vi "Check_Execution_Row.vi"(0 "Execution Row":T1 {"Carrier_2 Q (l/min)" format="%#.2f"; "Row Duration (mins)" format="%#.1f"; "Row No" min=0; "Trace Gas Concentration (%)" min=0.0 format="%#_4f"; "Carrier_1 Q (l/min)" format="%#.2f"; "Tunnel Speed" format="%#.2f"; "Start X" format="%#.2f"; "Start Y" format="%#.2f"; "Start Z" format="%#.2f"; "End X" format="%#.2f"; "End Y" format="%#.2f"; "End Z" format="%#.2f"; "Averaging time (min)" min=0.0 format="%#.2f"}, 1 "Earlier Filenames":path[](array[path]), 3 "Synchronization Start No":i32=1 min=1 max=100, 4 "Row Index":i32, 5 "Max Tunnel Speed":dbl format="%.2f") -> (6 "Edited Row":bool, 7 "Execution Row Out":T1 {"Carrier_2 Q (l/min)" format="%#.2f"; "Row Duration (mins)" format="%#.1f"; "Row No" min=0; "Trace Gas Concentration (%)" min=0.0 format="%#_4f"; "Carrier_1 Q (l/min)" format="%#.2f"; "Tunnel Speed" format="%#.2f"; "Start X" format="%#.2f"; "Start Y" format="%#.2f"; "Start Z" format="%#.2f"; "End X" format="%#.2f"; "End Y" format="%#.2f"; "End Z" format="%#.2f"; "Averaging time (min)" min=0.0 format="%#.2f"}, 9 "Continue?":bool, 10 "Error Comments":string)   [LabVIEW 2015]
uses:
  Traverse_cluster.ctl
  Spacing.ctl
  Controls/Multi_run_mode.ctl
  Controls/User_Specific_mode.ctl
  Controls/Home.ctl
  Controls/Tunnel_Coordinates.ctl
  ADAM Client/Sub VIs/ADAM Controls/Channel_names.ctl
  Globals/Extra_Commands_Global.vi
  Globals/Constants_global.vi
  Globals/Trav_pos_global.vi
panel:
  out "Traverse line Out":T1 {"Carrier_2 Q (l/min)" format="%#.2f"; "Row Duration (mins)" format="%#.1f"; "Row No" min=0; "Trace Gas Concentration (%)" min=0.0 format="%#_4f"; "Carrier_1 Q (l/min)" format="%#.2f"; "Tunnel Speed" format="%#.2f"; "Start X" format="%#.2f"; "Start Y" format="%#.2f"; "Start Z" format="%#.2f"; "End X" format="%#.2f"; "End Y" format="%#.2f"; "End Z" format="%#.2f"; "Averaging time (min)" min=0.0 format="%#.2f"}
  out "Fixed Axis":bool[](array[boolean])
  out "Filenames":string[](array[string])
  out "Current Sync Number":i32
  out "Checks":string[](array[string])
  in  "Edit in Excel":bool
  in  "OK":bool
  # "X           Y            Z"
  # "Start"
  # "End"
  # "X           Y            Z"
  # "Start"
  # "End"
  # "X           Y            Z"
  # "Start"
  # "End"
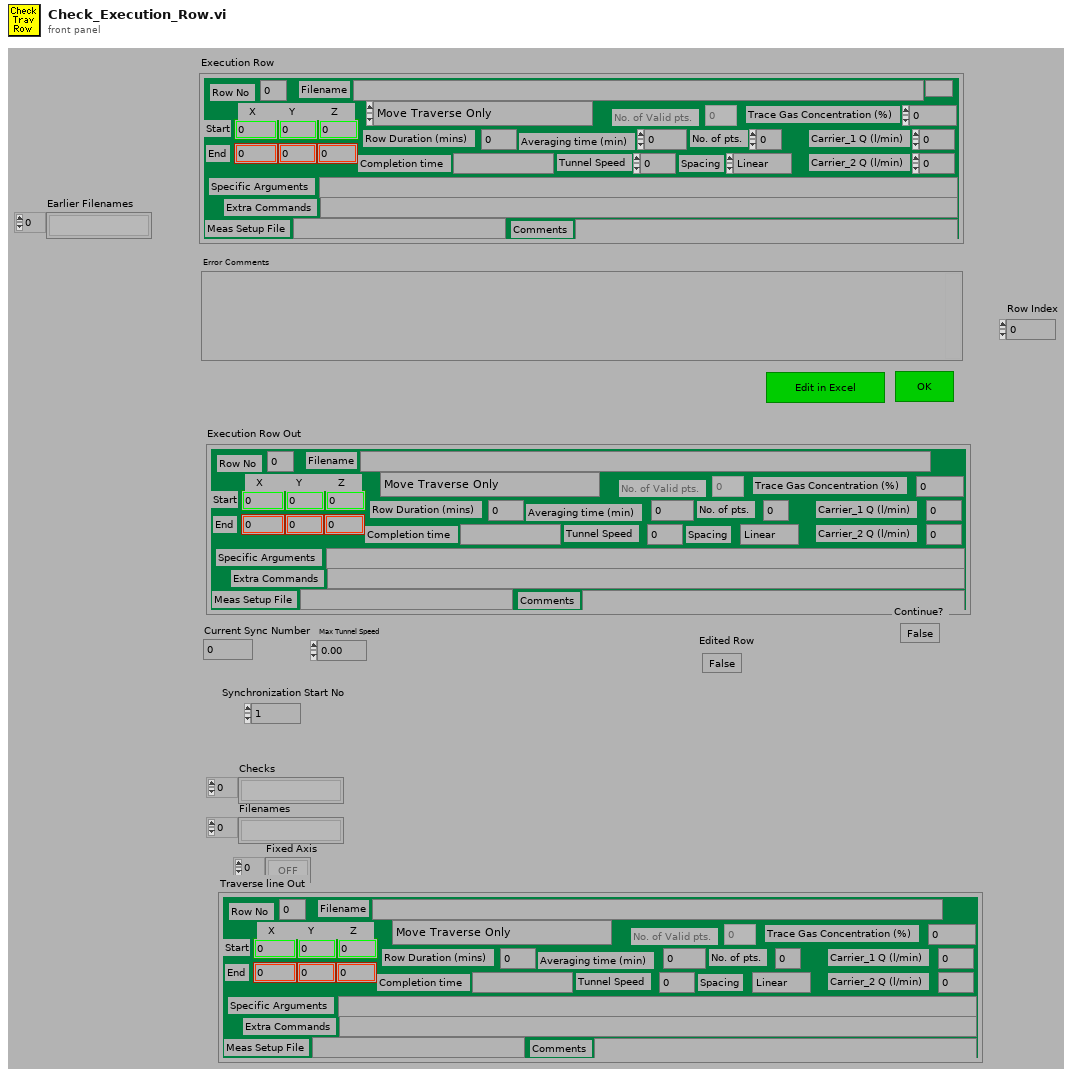
[diagram p1: front panel]
types:
  T1 = typedef "Traverse_cluster.ctl" = cluster{"Start X":sgl, "Start Y":sgl, "Start Z":sgl, "End X":sgl, "End Y":sgl, "End Z":sgl, "No. of pts.":i32, "Spacing":T2, "Filename":path, "Tunnel Speed":dbl, "Averaging time (min)":dbl, "Extra Commands":string, "Carrier_1 Q (l/min)":dbl, "Carrier_2 Q (l/min)":dbl, "Trace Gas Concentration (%)":dbl, "Specific Arguments":string, "Comments":string, "Row No":i32, "Row Type Selector":T3, "Completion time":string, "Row Duration (mins)":dbl, "No. of Valid pts.":i32, "Meas Setup File":string}
  T2 = typedef "Spacing.ctl" = enum16{"Linear", "Log", "Gauss", "Specified", "N/A"}
  T3 = typedef "Multi_run_mode.ctl" = enum16{"Move Traverse Only", "Set Tunnel Speed Only", "Set Source Only", "Set Measurement Conditions", "Single Measurement", "Vertical Profile", "Lateral Profile", "Longitudinal Profile", "Explore Volume", "Multi-Axis Profile", "Auto Calibrate", "Meas Fast FID Bkgnd", "Check Beam Power", "Scanning Valve Measurement", "Run VI Named:", "Set ADAM Ch", "Wait (minutes)", "Send Message", "Synchronize With:", "Fall Back to this Row", "Turn Off Row Repeating", "Blank Row", "Traverse 3D Volume"}
  T4 = enum16{"All Channel Names", "Valid Channel Names"}
  T5 = typedef "User_Specific_mode.ctl" = enum16{"Check VI only", "Run VI"}
  T6 = typedef "Home.ctl" = enum16{"Don't Home", "Home  +X", "Home  -X", "Home  +Y", "Home  -Y", "Home  +Z", "Home  -Z"}
  T7 = typedef "Tunnel_Coordinates.ctl" = enum16{"Work in Tunnel Coordinates", "Work in Model Coordinates"}
  T8 = enum16{"Zero or one", "One", "Zero or more", "One or more"}
  T9 = typedef "Channel_names.ctl" = enum16{"Active Only", "Active + Off", "All Channels"}
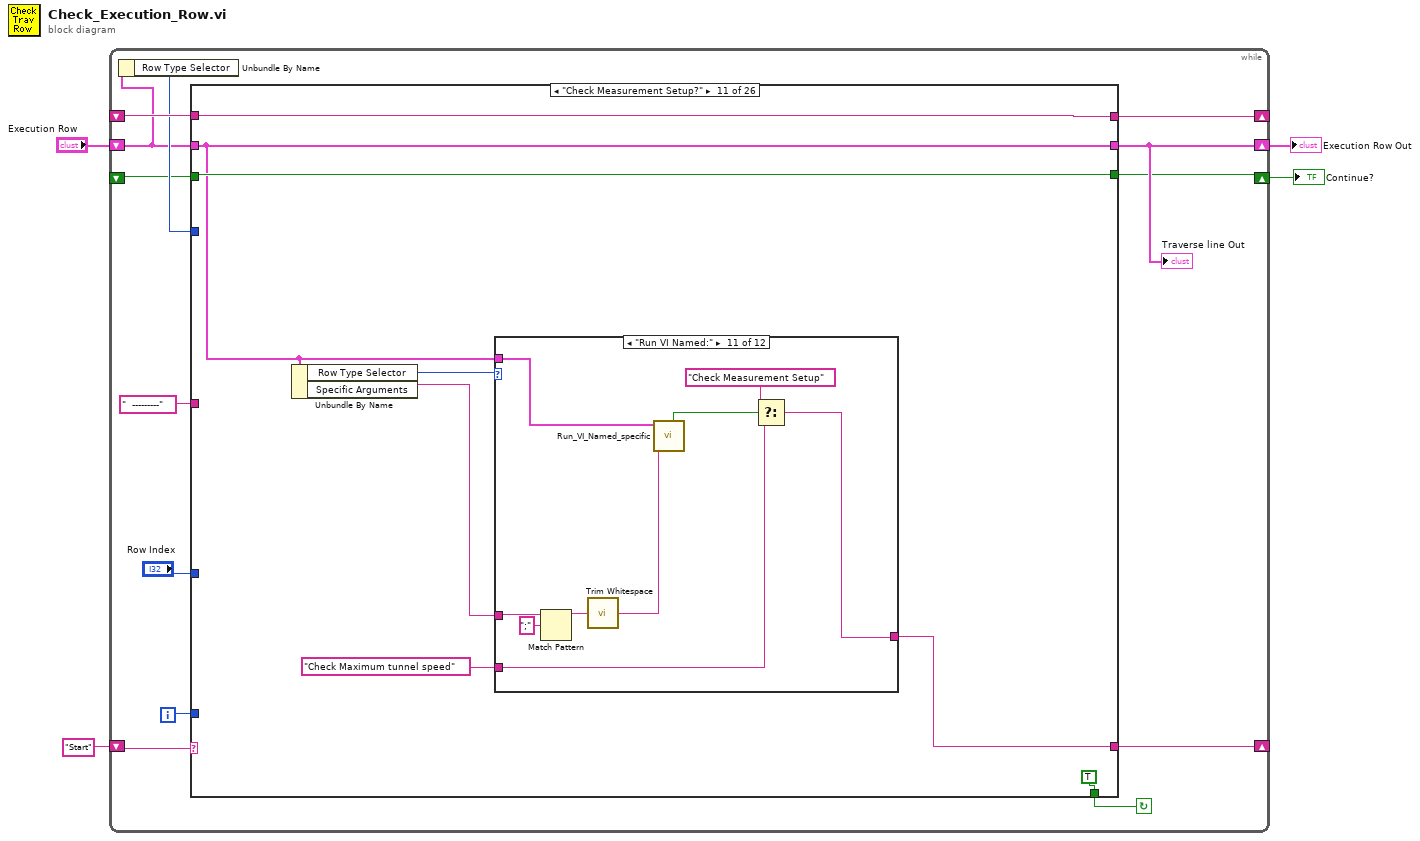
[diagram p0: block diagram]
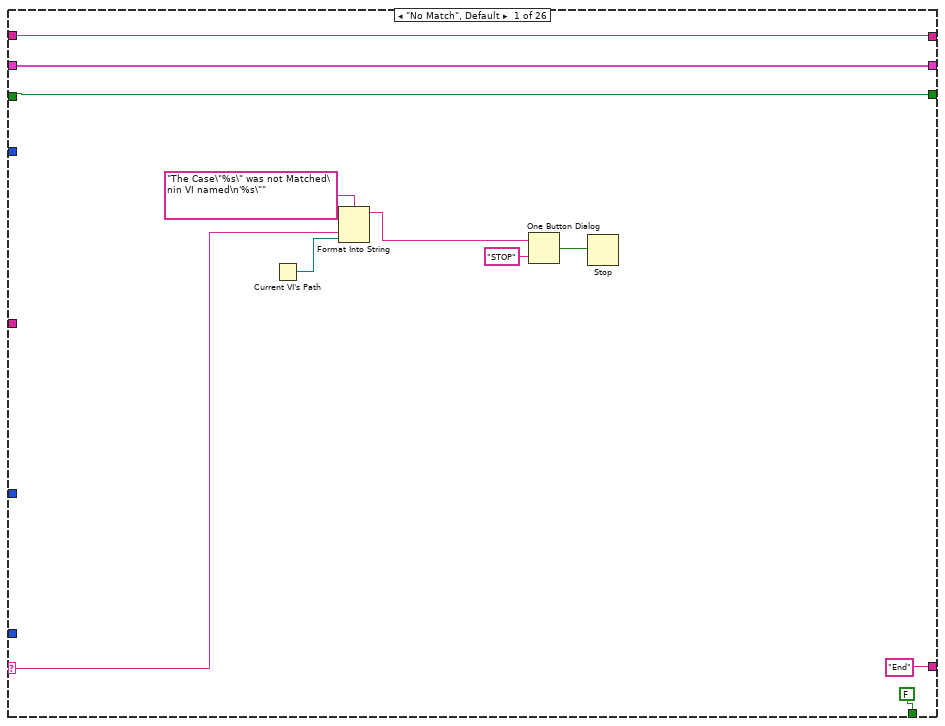
[diagram p2: hidden frame]
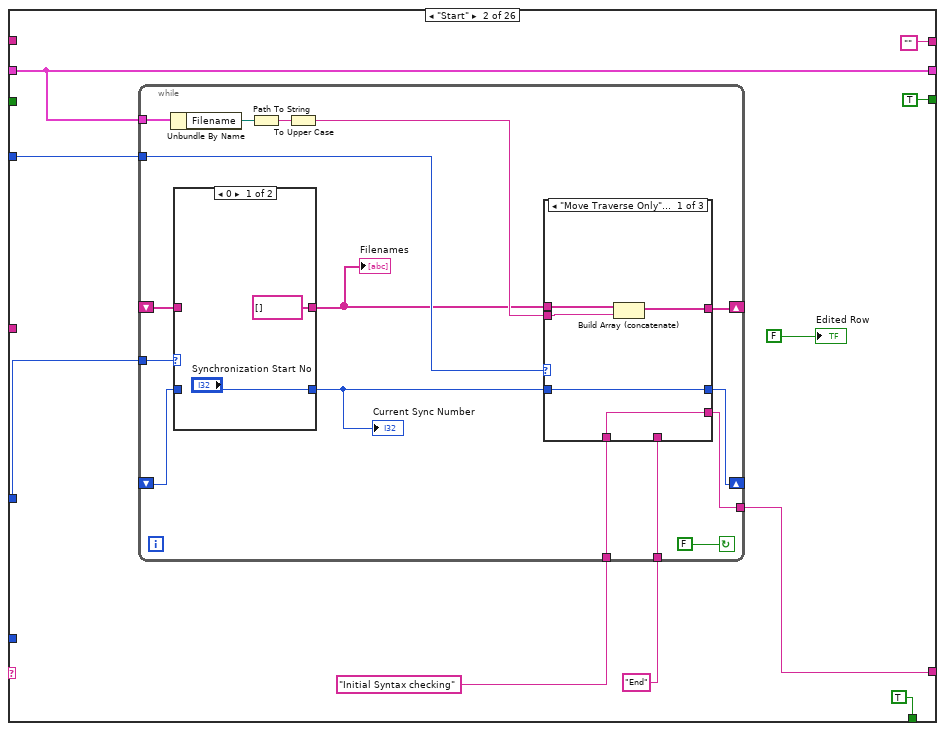
[diagram p3: hidden frame]
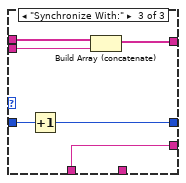
[diagram p6: hidden frame]
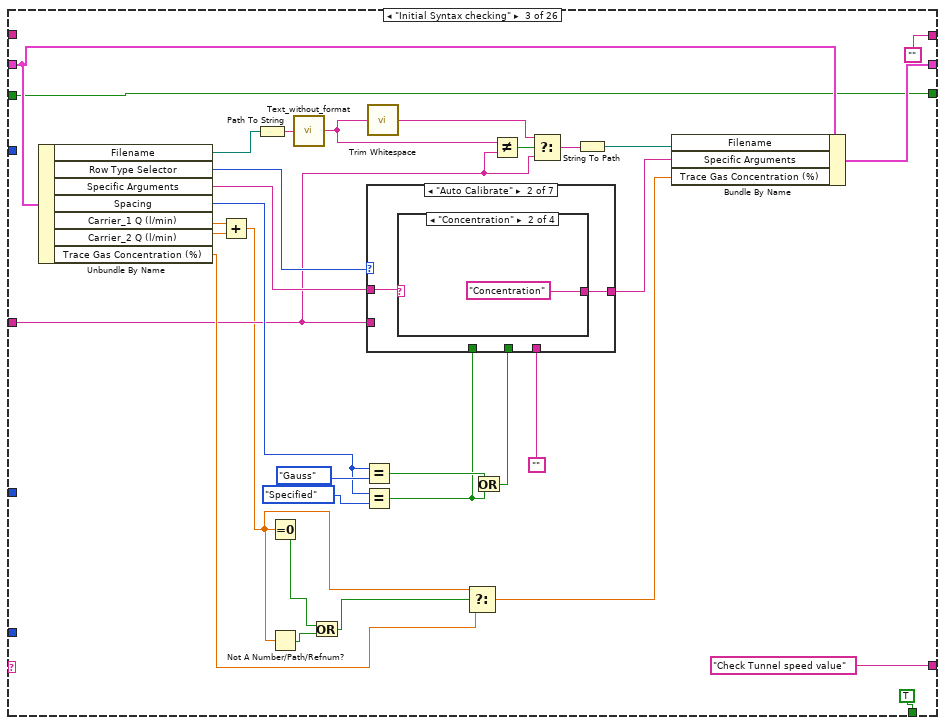
[diagram p7: hidden frame]
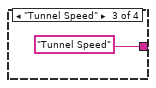
[diagram p10: hidden frame]
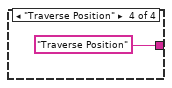
[diagram p11: hidden frame]
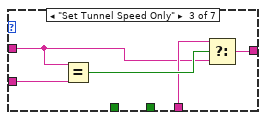
[diagram p12: hidden frame]
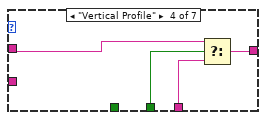
[diagram p13: hidden frame]
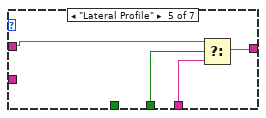
[diagram p14: hidden frame]
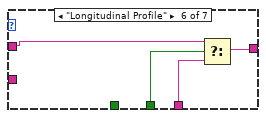
[diagram p15: hidden frame]
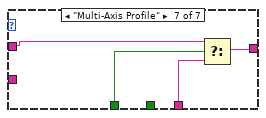
[diagram p16: hidden frame]
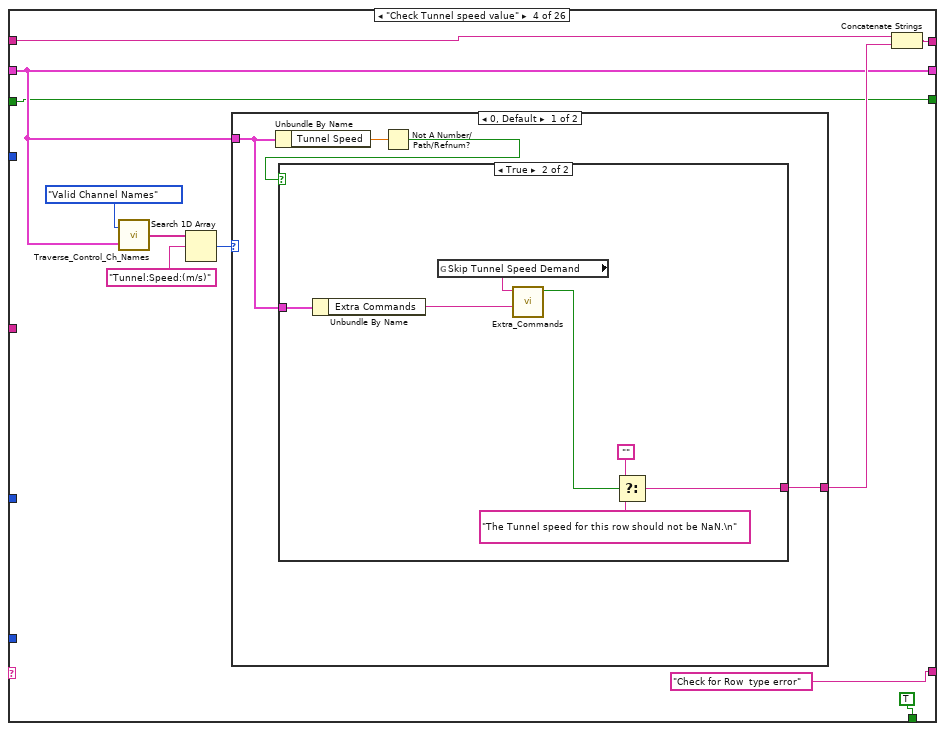
[diagram p17: hidden frame]
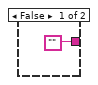
[diagram p18: hidden frame]
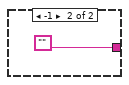
[diagram p19: hidden frame]
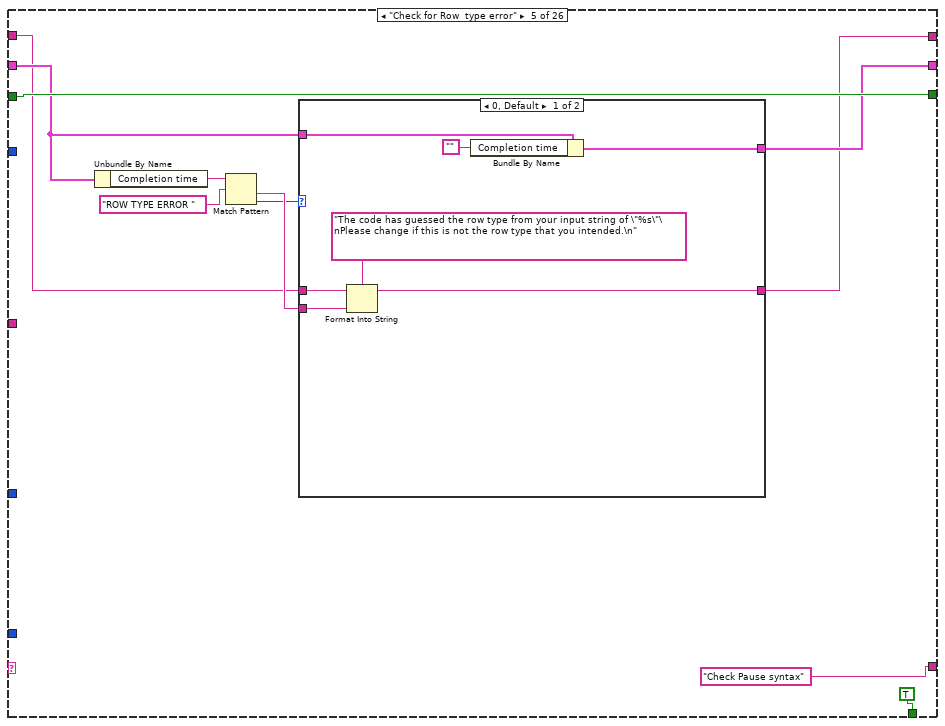
[diagram p20: hidden frame]
diagram:
  n1 = while {
    shift-left: _ -> [w16]
    shift-right: [w17] -> _
    shift-left: "Start" -> [w9]
    shift-right: [w14] -> _
    shift-right: [w8] -> w2
    shift-left: "Execution Row" -> [w5]
    shift-right: [w7] -> w1
    shift-left: _ -> [w6]
    i -> [w10]
    stop <- w15 continue-if-true
    n2 = Unbundle By Name(w5) -> ("Row Type Selector"=w12:T3)
    n3 = case shown="\"Check Measurement Setup?\"" w9 {
      tunnel: w5 -> [w23 w32 w99 w136 w160 w192 w217 w268 w315 w341 w397 w429 w437 w476 w846 w946 w983 w1011 w1093 w1104 w1112 w1180 _ w1217 w1224 w1234]
      tunnel: "  ---------" ("f") -> [_ _ w77 _ _ w196 _ _ _ _ _ _ _ _ _ _ _ _ _ _ _ _ _ _ _ _]
      tunnel: "Row Index" -> [_ w36 _ _ _ _ w214 _ _ _ _ _ _ w470 _ _ _ _ _ _ _ _ _ w1218 _ w1233]
      selector: w9 -> [w18 _ _ _ _ _ _ _ _ _ _ _ _ _ _ _ _ _ _ _ _ _ _ _ _ _]
      tunnel: [w22 "" "" w137 w157 w185 w223 w273 w320 w346 w399 w433 w442 w480 w851 w956 w989 w1034 w1092 w1106 w1113 w1186 w1195 w1219 w1229 w1236] -> w17
      tunnel: w12 -> [_ w35 _ _ _ w178 _ _ _ _ _ _ w440 w479 w847 w944 _ _ _ _ w1117 _ _ _ _ _]
      tunnel: w16 -> [w22 _ _ w138 w158 w187 w224 w274 w321 w347 w399 w432 w443 w481 w851 w957 w990 w1035 w1092 w1107 w1118 w1186 w1195 w1219 w1229 w1236]
      tunnel: [FALSE TRUE TRUE TRUE TRUE TRUE TRUE TRUE TRUE TRUE TRUE TRUE TRUE TRUE TRUE TRUE TRUE TRUE TRUE TRUE w1109 TRUE TRUE TRUE TRUE FALSE] -> w15
      tunnel: ["End" w33 "Check Tunnel speed value" ("f") "Check for Row  type error" ("f") "Check Pause syntax" ("f") w190 "Check Traverse Setup Name" ("f") "Check Datum Image Extra command" ("f") "Check IF command" ("f") "Check Measurement Setup?" ("f") w401 "Check Maximum tunnel speed" ("f") "Row type specific check" ("f") w477 "Check for position NaNs" ("f") w947 "Check source details" ("t") "Check source details" ("f") w1089 "check entered filename etc" ("f") w1115 "What to do next?" ("f") w1193 "Initial Syntax checking" "End" "End"] -> w14
      tunnel: w10 -> [_ _ _ _ _ _ _ _ _ _ _ _ _ _ _ _ _ _ _ _ _ _ _ _ _ _]
      tunnel: [w23 w32 w80 w136 w161 w180 w216 w268 w315 w341 w397 w428 w437 w471 w845 w946 w983 w1010 w1093 w1104 w1111 w1180 w1188 w1220 w1224 w1232] -> w8
      tunnel: [w19 TRUE w78 w135 w167 w181 w218 w266 w313 w338 w403 w430 w435 w473 w843 w945 w982 w1008 w1094 w1102 w1109 w1179 w1187 w1214 w1223 w1230] -> w7
      tunnel: w6 -> [w19 _ w78 w135 w167 w181 w218 w266 w313 w338 w403 w430 w435 w473 w843 w945 w982 w1008 w1094 w1102 _ w1179 _ w1214 w1223 w1230]
      frame "No Match", Default {
        n4 = Current VI's Path() -> (path=w24:path)
        n5 = Format Into String(format string="The Case\"%s\" was not Matched\nin VI named\n'%s\"" ("Format String"), w18, w24) -> (resulting string=w27:string)  [unwired: 2 in, 1 out]
        n6 = One Button Dialog(message=w27, button name ("OK")="STOP") -> (true=w25:bool)
        n7 = Stop(stop? (T)=w25) -> ()
      }
      frame "Start" {
        n8 = while {
          tunnel: "End" -> [w40]
          tunnel: "Initial Syntax checking" -> [w41]
          tunnel: [w42] -> w33
          tunnel: w32 -> [w49]
          shift-left: _ -> [w48]
          shift-right: [w47] -> _
          tunnel: w35 -> [w53]
          shift-left: _ -> [w52]
          shift-right: [w51] -> _
          tunnel: w36 -> [w54]
          stop <- FALSE continue-if-true
          n9 = Unbundle By Name(w49) -> ("Filename"=w46:path)
          n10 = case shown="0" w54 {
            tunnel: ["Synchronization Start No" w58] -> w50
            tunnel: w52 -> [_ w58]
            tunnel: w48 -> [_ w57]
            tunnel: [string[] [] w57] -> w43
            frame 0 {
            }
            frame 1, Default {
            }
          }
          "Current Sync Number" <- w50
          "Filenames" <- w43
          n11 = Path To String(path=w46) -> (string=w45:string)
          n12 = To Upper Case(1:w45) -> (0:w44:string)
          n13 = case shown="\"Move Traverse Only\", Default" w53 {
            tunnel: w50 -> [w63 w66 w72]
            tunnel: [w63 w66 w71] -> w51
            tunnel: w44 -> [w61 _ w70]
            tunnel: w43 -> [w62 w65 w69]
            tunnel: [w60 w65 w68] -> w47
            tunnel: [w59 w64 w67] -> w42
            tunnel: w41 -> [w59 _ w67]
            tunnel: w40 -> [_ w64 _]
            frame "Move Traverse Only", Default {
              n14 = Build Array (concatenate)(w62, w61) -> (w60:string[])
            }
            frame "Blank Row" {
            }
            frame "Synchronize With:" {
              n15 = Increment(x=w72) -> (x+1=w71:i32)
              n16 = Build Array (concatenate)(w69, w70) -> (w68:string[])
            }
          }
        }
        "Edited Row" <- FALSE ("Editted Row")
      }
      frame "Initial Syntax checking" {
        n17 = Unbundle By Name(w99) -> ("Filename"=w76:path, "Row Type Selector"=w97:T3, "Specific Arguments"=w95:string, "Spacing"=w87:T2, "Carrier_1 Q (l/min)"=w75:dbl, "Carrier_2 Q (l/min)"=w74:dbl, "Trace Gas Concentration (%)"=w93:dbl)
        n18 = Add(x=w75, y=w74) -> (x+y=w73:dbl)
        n19 = Path To String(path=w76) -> (string=w82:string)
        n20 = Equal To 0?(x=w73) -> (x = 0?=w85:bool)
        n21 = Not A Number/Path/Refnum?(number/path/refnum=w73) -> (NaN/Path/Refnum?=w84:bool)
        n22 = call "Text_without_format.vi"("Input string"=w82) -> ("Output string"=w103:string)
        n23 = Or(x=w85, y=w84) -> (x .or. y?=w83:bool)
        n24 = Equal?(x=w87, y=Spacing."Gauss" ("Spacing")) -> (x = y?=w89:bool)
        n25 = Equal?(x=w87, y=Spacing."Specified" ("Spacing")) -> (x = y?=w86:bool)
        n26 = call <vilib>:"Trim Whitespace.vi"("string"=w103) -> ("trimmed string"=w102:string)  [unwired: 1 in]
        n27 = Select(t=w73, s=w83, f=w93) -> (s? t:f=w92:dbl)
        n28 = Or(x=w89, y=w86) -> (x .or. y?=w88:bool)
        n29 = case shown="\"Auto Calibrate\"" w97 {
          tunnel: [w105 w107 w112 w118 w122 w126 w130] -> w96
          tunnel: w95 -> [w105 w106 w113 w120 w124 w128 w132]
          tunnel: "" -> [_ _ w114 w119 w123 w127 w131]
          tunnel: w88 -> [_ _ _ w117 w121 w125 _]
          tunnel: w86 -> [_ _ _ _ _ _ w129]
          tunnel: w77 -> [_ _ w116 _ _ _ _]
          frame "Move Traverse Only", Default {
          }
          frame "Auto Calibrate" {
            n30 = case shown="\"Concentration\"" w106 {
              selector: w106 -> [w108 _ _ _]
              tunnel: [w108 "Concentration" "Tunnel Speed" "Traverse Position"] -> w107
              frame "No Match", Default {
              }
              frame "Concentration" {
              }
              frame "Tunnel Speed" {
              }
              frame "Traverse Position" {
              }
            }
          }
          frame "Set Tunnel Speed Only" {
            n31 = Equal?(x=w113, y=w116) -> (x = y?=w115:bool)
            n32 = Select(t=w114, s=w115, f=w113) -> (s? t:f=w112:string)
          }
          frame "Vertical Profile" {
            n33 = Select(t=w120, s=w117, f=w119) -> (s? t:f=w118:string)
          }
          frame "Lateral Profile" {
            n34 = Select(t=w124, s=w121, f=w123) -> (s? t:f=w122:string)
          }
          frame "Longitudinal Profile" {
            n35 = Select(t=w128, s=w125, f=w127) -> (s? t:f=w126:string)
          }
          frame "Multi-Axis Profile" {
            n36 = Select(t=w132, s=w129, f=w131) -> (s? t:f=w130:string)
          }
        }
        n37 = Not Equal?(x=w103, y=w77) -> (x != y?=w104:bool)
        n38 = Select(t=w102, s=w104, f=w77) -> (s? t:f=w101:string)
        n39 = String To Path(string=w101) -> (path=w81:path)
        n40 = Bundle By Name(cluster=w99, "Filename"=w81, "Specific Arguments"=w96, "Trace Gas Concentration (%)"=w92) -> (w80:T1)
      }
      frame "Check Tunnel speed value" {
        n41 = call "Traverse_Control_Ch_Names.vi"("Traverse line"=w136, "Mode"=T4."Valid Channel Names") -> ("Channel names"=w142:string[])
        n42 = Search 1D Array(1D array=w142, element="Tunnel:Speed:(m/s)" ("Label for value")) -> (index of element=w140:i32)  [unwired: 1 out]
        n43 = case shown="0, Default" w140 {
          tunnel: w136 -> [w145 _]
          tunnel: [w144 ""] -> w139
          frame 0, Default {
            n44 = Unbundle By Name(w145) -> ("Tunnel Speed"=w147:dbl)
            n45 = Not A Number/Path/Refnum?(number/path/refnum=w147) -> (NaN/Path/Refnum?=w146:bool)
            n46 = case shown="True" w146 {
              tunnel: w145 -> [_ w155]
              tunnel: ["" w149] -> w144
              frame False {
              }
              frame True {
                n47 = Unbundle By Name(w155) -> ("Extra Commands"=w153:string)
                n48 = global read "Extra_Commands_Global.vi" "Skip Tunnel Speed Demand"() -> (w154:string)
                n49 = call "Extra_Commands.vi"("String to Search"=w153, "Command"=w154) -> ("Command Found"=w152:bool)  [unwired: 1 in, 4 out]
                n50 = Select(t="", s=w152, f="The Tunnel speed for this row should not be NaN.\n") -> (s? t:f=w149:string)
              }
            }
          }
          frame -1 {
          }
        }
        n51 = Concatenate Strings(w138, w139) -> (w137:string)
      }
      frame "Check for Row  type error" {
        n52 = Unbundle By Name(w160) -> ("Completion time"=w163:string)
        n53 = Match Pattern(string=w163, regular expression="ROW TYPE ERROR " ("format string")) -> (after substring=w162:string, offset past match=w159:i32)  [unwired: 3 out]
        n54 = case shown="0, Default" w159 {
          tunnel: w162 -> [w174 _]
          tunnel: [w172 w176] -> w161
          tunnel: w160 -> [w171 w176]
          tunnel: [w169 w175] -> w157
          tunnel: w158 -> [w168 w175]
          frame 0, Default {
            n55 = Format Into String(format string="The code has guessed the row type from your input string of \"%s\"\nPlease change if this is not the row type that you intended.\n", initial string=w168, w174) -> (resulting string=w169:string)  [unwired: 1 in, 1 out]
            n56 = Bundle By Name(cluster=w171, "Completion time"="") -> (w172:T1)
          }
          frame -1 {
          }
        }
      }
      frame "Check Pause syntax" {
        n57 = Unbundle By Name(w192) -> ("Extra Commands"=w197:string)
        n58 = Equal?(x=Multi_run_mode."Set ADAM Ch" ("Row Type Selector"), y=w178) -> (x = y?=w177:bool)
        n59 = Not Equal?(x=w197, y=w196) -> (x != y?=w198:bool)
        n60 = Select(t=w197, s=w198, f="") -> (s? t:f=w194:string)
        n61 = call <vilib>:"Trim Whitespace.vi"("string"=w194) -> ("trimmed string"=w189:string)  [unwired: 1 in]
        n62 = case shown="False" w177 {
          tunnel: [w200 TRUE] -> w191
          tunnel: w189 -> [w199 _]
          frame False {
            n63 = Equal?(x=w199, y="") -> (x = y?=w200:bool)
          }
          frame True {
          }
        }
        n64 = call "Pause_for_server_ch_val.vi"("Extra command string"=w189, "Simulate/Run"=User_Specific_mode."Check VI only") -> ("Extra command string Out"=w188:string, "Error Comments"=w186:string)
        n65 = Bundle By Name(cluster=w192, "Extra Commands"=w188) -> (w180:T1)
        n66 = Concatenate Strings(w187, w186) -> (w185:string)
        n67 = Select(t="Check Measurement Setup?", s=w191, f="Check Extra Commands") -> (s? t:f=w190:string)
      }
      frame "Check Extra Commands" {
        n68 = global read "Extra_Commands_Global.vi" "Home"() -> (w203:string)
        n69 = Unbundle By Name(w217) -> ("Extra Commands"=w209:string)
        n70 = for {
          N: 4 -> [_]
          tunnel: w209 -> [w242]
          shift-right: [w238] -> w204
          shift-left: "" -> [w239]
          i -> [w244]
          n71 = case shown="0, Default" w244 {
            tunnel: [w247 w249 w251 w253] -> w241
            tunnel: ["The Extra Command \"%s\" should have a numeric argument of (Centre; Intensity) eg 0 ; 0.85 for Gaussian spacing or (Offset) eg 300 for Log \n" ("Format String") "The Extra Command \"%s\" should have a numeric argument.\n" ("Format String") "The Extra Command \"%s\" should have a numeric argument.\n" ("Format String") "The Extra Command \"%s\" should have a numeric argument greater than Zero.\n" ("Format String")] -> w236
            frame 0, Default {
              n72 = global read "Extra_Commands_Global.vi" "Point Spacing Parameters"() -> (w247:string)
            }
            frame 1 {
              n73 = global read "Extra_Commands_Global.vi" "Establish Exp Conditions (s)"() -> (w249:string)
            }
            frame 2 {
              n74 = global read "Extra_Commands_Global.vi" "Minutes Before Repeating Row"() -> (w251:string)
            }
            frame 3 {
              n75 = global read "Extra_Commands_Global.vi" "Puff Duration Sec"() -> (w253:string)
            }
          }
          n76 = call "Extra_Commands.vi"("String to Search"=w242, "Command"=w241) -> ("String Value"=w243:string, "Command Found"=w245:bool)  [unwired: 1 in, 3 out]
          n77 = case shown="True" w245 {
            tunnel: w243 -> [_ w262]
            tunnel: w241 -> [_ w260]
            tunnel: [w254 w257] -> w240
            tunnel: "" -> [w254 w256]
            tunnel: w236 -> [_ w255]
            frame False {
            }
            frame True {
              n78 = Decimal String To Number(string=w262) -> (offset past number=w261:i32)  [unwired: 3 out]
              n79 = Equal To 0?(x=w261) -> (x = 0?=w259:bool)
              n80 = Format Into String(format string=w255, w260) -> (resulting string=w258:string)  [unwired: 2 in, 1 out]
              n81 = Select(t=w258, s=w259, f=w256) -> (s? t:f=w257:string)
            }
          }
          n82 = Concatenate Strings(w240, w239) -> (w238:string)
        }
        n83 = call "Extra_Commands.vi"("String to Search"=w209, "Command"=w203) -> ("String Value"=w207:string, "Command Found"=w208:bool)  [unwired: 1 in, 3 out]
        n84 = case shown="True" w208 {
          tunnel: w207 -> [_ w235]
          tunnel: [TRUE w232] -> w206
          frame False {
          }
          frame True {
            n85 = call "Home_String_to_Enumerated_Type.vi"("String"=w235) -> ("Home"=w234:T6)
            n86 = Not Equal?(x=w234, y=Home."Don't Home" ("Home")) -> (x != y?=w232:bool)
          }
        }
        n87 = call "Trav_Prog_Extra_Commands.vi"() -> ("Extra Commands Array"=w219:string[])  [unwired: 2 out]
        n88 = call "Valid_Extra_Command.vi"("Extra Commands string"=w209, "Valid Commands Array"=w219) -> ("Output String"=w222:string, "Extra Commands string Out"=w215:string)  [unwired: 3 out]
        n89 = Bundle By Name(cluster=w217, "Extra Commands"=w215) -> (w216:T1)
        n90 = call "Skip_If Sd_Error_Below.vi"("String to Search"=w215, "Simulate/Run"=User_Specific_mode."Check VI only", "Measurement setup Applied?"=FALSE, "Row Number"=w214) -> ("Error String"=w211:string)  [unwired: 1 in, 4 out]
        n91 = case shown="False" w206 {
          tunnel: [w228 w230] -> w205
          tunnel: w204 -> [w227 w230]
          tunnel: w203 -> [w229 _]
          frame False {
            n92 = Format Into String(format string="The Extra Command \"%s\" argument should be either\nHome  +X\nHome  -X\nHome  +Y\nHome  -Y\nHome  +Z\nHome  -Z\n" ("Format String"), initial string=w227, w229) -> (resulting string=w228:string)  [unwired: 1 in, 1 out]
          }
          frame True {
          }
        }
        n93 = Concatenate Strings(w224, w222, w205, w211) -> (w223:string)
      }
      frame "Check Traverse Setup Name" {
        n94 = Unbundle By Name(w268) -> ("Extra Commands"=w265:string)
        n95 = global read "Extra_Commands_Global.vi" "!Traverse Setup"() -> (w271:string)
        n96 = call "Extra_Commands.vi"("String to Search"=w265, "Command"=w271) -> ("String Value"=w269:string, "Command Found"=w270:bool)  [unwired: 1 in, 3 out]
        n97 = case shown="True" w270 {
          tunnel: w269 -> [_ w285]
          tunnel: [w275 w281] -> w267
          tunnel: "" -> [w275 w280]
          frame False {
          }
          frame True {
            n98 = call "Get_array_values_fr_String.vi"("String Value"=w285) -> ("String array"=w277:string[])  [unwired: 1 out]
            n99 = global read "Constants_global.vi" "Traverse folder"() -> (w286:path)
            n100 = Empty Array?(array=w277) -> (empty?=w278:bool)
            n101 = Select(t=string[] [""], s=w278, f=w277) -> (s? t:f=w279:string[])
            n102 = List Folder(path=w286) -> (folder names=w283:string[])  [unwired: 1 in, 5 out]
            n103 = for {
              tunnel: w279 -> [w302] mode=indexing
              tunnel: w283 -> [w304]
              shift-right: [w300] -> w284
              shift-left: w280 -> [w301]
              n104 = Search 1D Array(1D array=w304, element=w302) -> (index of element=w303:i32)  [unwired: 1 out]
              n105 = case shown="-1" w303 {
                tunnel: w302 -> [_ w308]
                tunnel: [w305 w307] -> w300
                tunnel: w301 -> [w305 w306]
                frame Default {
                }
                frame -1 {
                  n106 = Format Into String(format string="%s is not a valid Travese setup.\n", initial string=w306, w308) -> (resulting string=w307:string)  [unwired: 1 in, 1 out]
                }
              }
            }
            n107 = Empty String/Path?(string/path=w284) -> (empty?=w282:bool)
            n108 = case shown="False" w282 {
              tunnel: w283 -> [w293 _]
              tunnel: [w292 w299] -> w281
              tunnel: w284 -> [w290 w299]
              frame False {
                w287 = "\r\n"
                n109 = Concatenate Strings(w290, " Valid option are:" ("format string"), w287) -> (w289:string)
                n110 = for {
                  shift-right: [w296] -> w292
                  shift-left: w289 -> [w297]
                  tunnel: w293 -> [w298] mode=indexing
                  tunnel: "!Traverse Setup =  " ("Substring") -> [w295]
                  tunnel: w287 -> [w294]
                  n111 = Concatenate Strings(w297, w295, w298, w294) -> (w296:string)
                }
              }
              frame True {
              }
            }
          }
        }
        n112 = Concatenate Strings(w274, w267) -> (w273:string)
      }
      frame "Check Datum Image Extra command" {
        n113 = Unbundle By Name(w315) -> ("Extra Commands"=w312:string)
        n114 = global read "Extra_Commands_Global.vi" "Datum Image"() -> (w318:string)
        n115 = call "Extra_Commands.vi"("String to Search"=w312, "Command"=w318) -> ("String Value"=w316:string, "Command Found"=w317:bool)  [unwired: 1 in, 3 out]
        n116 = case shown="True" w317 {
          tunnel: w316 -> [_ w328]
          tunnel: [w322 w325] -> w314
          tunnel: "" -> [w322 w324]
          frame False {
          }
          frame True {
            n117 = Build Path(base path=path "hello", name or relative path=w328) -> (appended path=w327:path)
            n118 = call "Current_Filepath.vi"("Short_Name"="Cal" ("Data Type"), "Filename in"=w327, "Data Type"="Calibrations") -> ("Filename Out"=w323:path)  [unwired: 1 in, 1 out]
            n119 = call "Does_file_exist_(simple).vi"("Pathname"=w323) -> ("exists?"=w326:bool)
            n120 = case shown="False" w326 {
              tunnel: [w332 w335] -> w325
              tunnel: w324 -> [_ w335]
              tunnel: w323 -> [w334 _]
              frame False {
                n121 = Format Into String(format string="Cannot find Datum Image File\n%s", w334) -> (resulting string=w332:string)  [unwired: 2 in, 1 out]
              }
              frame True {
              }
            }
          }
        }
        n122 = Concatenate Strings(w321, w314) -> (w320:string)
      }
      frame "Check IF command" {
        n123 = Unbundle By Name(w341) -> ("Extra Commands"=w337:string)
        n124 = global read "Extra_Commands_Global.vi" "If Command"() -> (w344:string)
        n125 = call "Extra_Commands.vi"("String to Search"=w337, "Command"=w344) -> ("String Value"=w342:string, "Command Found"=w343:bool)  [unwired: 1 in, 3 out]
        n126 = case shown="True" w343 {
          tunnel: w342 -> [_ w353]
          tunnel: [w348 w352] -> w339
          tunnel: "" -> [w348 w350]
          frame False {
          }
          frame True {
            n127 = call "Get_array_values_fr_String.vi"("String Value"=w353) -> ("Numeric Array"=w349:dbl[], "String array"=w351:string[])
            n128 = Index Array(array=w351, index=0 ("Index")) -> (element=w354:string)
            n129 = case shown="\"Global Value Between\"" w354 {
              tunnel: w353 -> [w359 _ _ _]
              tunnel: [w358 w384 w385 "The !If  command has not been recognised.\nExtra command Example:\n!IF = Time Between;10:45;and;14:00;Execute Row (or) Skip Row\n\n!IF = ADAM Channel Between;Channel Name; 0.5;1.0\n\n!IF = Global Value Between; 0.5;1.0" ("Error Comments")] -> w352
              tunnel: w351 -> [_ w375 w393 _]
              tunnel: w350 -> [_ w368 w386 _]
              tunnel: w349 -> [_ _ _ _]
              frame "Time Between" {
                n130 = Get Date/Time In Seconds() -> (seconds since 1Jan1904=w356:timestamp)
                n131 = To Double Precision Float(number=w356) -> (double precision float=w357:dbl)
                n132 = call "If_Time_arguments.vi"("seconds since 1Jan1904"=w357, "String Value"=w359) -> ("Error Comments"=w358:string)  [unwired: 2 out]
              }
              frame "ADAM Channel Between" {
                n133 = Index Array(array=w375, index=1 ("Index")) -> (element=w378:string)
                n134 = Index Array(array=w375, index=2 ("Index")) -> (element=w374:string)
                n135 = Index Array(array=w375, index=3 ("Index")) -> (element=w373:string)
                n136 = Build Array(w378) -> (w380:string[])
                n137 = Decimal Digit?(1:w374) -> (0:w371:bool)
                n138 = Decimal Digit?(1:w373) -> (0:w372:bool)
                n139 = call "Get_Current_Scan_client.vi"("ADAM Ch Names"=w380) -> ("Numerical Values"=w382:dbl[])  [unwired: 3 out]
                n140 = And(x=w371, y=w372) -> (x .and. y?=w370:bool)
                n141 = Index Array(array=w382, index=0 ("Index")) -> (element=w383:dbl)
                n142 = Select(t=w368, s=w370, f="you must give two limits\n") -> (s? t:f=w364:string)
                n143 = Not A Number/Path/Refnum?(number/path/refnum=w383) -> (NaN/Path/Refnum?=w367:bool)
                n144 = Select(t="Invalid ADAM Channel Name\n", s=w367, f=w368) -> (s? t:f=w365:string)
                n145 = Concatenate Strings(w365, w364) -> (w362:string)
                n146 = Concatenate Strings(w362, "Extra command Example:\n!IF = ADAM Channel Between;Channel Name; 0.5;1.0") -> (w361:string)
                n147 = Empty String/Path?(string/path=w362) -> (empty?=w363:bool)
                n148 = Select(t=w368, s=w363, f=w361) -> (s? t:f=w384:string)
              }
              frame "Global Value Between" {
                n149 = Index Array(array=w393, index=1 ("Index")) -> (element=w392:string)
                n150 = Index Array(array=w393, index=2 ("Index")) -> (element=w391:string)
                n151 = Decimal Digit?(1:w392) -> (0:w389:bool)
                n152 = Decimal Digit?(1:w391) -> (0:w390:bool)
                n153 = And(x=w389, y=w390) -> (x .and. y?=w388:bool)
                n154 = Select(t=w386, s=w388, f="The Extra command IF statement must have two numerical values for the limits\n\nExtra command Example:\n!IF = Global Value Between; 0.5;1.0") -> (s? t:f=w385:string)
              }
              frame "No Match", Default {
              }
            }
          }
        }
        n155 = Concatenate Strings(w347, w339) -> (w346:string)
      }
      frame "Check Measurement Setup?" {
        n156 = Unbundle By Name(w397) -> ("Row Type Selector"=w402:T3, "Specific Arguments"=w400:string)
        n157 = case shown="\"Run VI Named:\"" w402 {
          tunnel: ["Check Measurement Setup" ("t") "Check Measurement Setup" ("t") "Check Measurement Setup" ("t") "Check Measurement Setup" ("t") "Check Measurement Setup" ("t") "Check Measurement Setup" ("t") "Check Measurement Setup" ("t") "Check Measurement Setup" ("t") "Check Measurement Setup" ("t") "Check Measurement Setup" ("t") w415 w424] -> w401
          tunnel: w400 -> [_ _ _ _ _ _ _ _ _ _ w422 _]
          tunnel: "Check Maximum tunnel speed" ("f") -> [_ _ _ _ _ _ _ _ _ _ w416 w424]
          tunnel: w397 -> [_ _ _ _ _ _ _ _ _ _ w419 _]
          frame "Lateral Profile" {
          }
          frame "Traverse 3D Volume" {
          }
          frame "Longitudinal Profile" {
          }
          frame "Explore Volume" {
          }
          frame "Multi-Axis Profile" {
          }
          frame "Vertical Profile" {
          }
          frame "Single Measurement" {
          }
          frame "Scanning Valve Measurement" {
          }
          frame "Auto Calibrate" {
          }
          frame "Meas Fast FID Bkgnd" {
          }
          frame "Run VI Named:" {
            n158 = Match Pattern(string=w422, regular expression=";") -> (before substring=w421:string)  [unwired: 4 out]
            n159 = call <vilib>:"Trim Whitespace.vi"("string"=w421) -> ("trimmed string"=w420:string)  [unwired: 1 in]
            n160 = call "Run_VI_Named_specific.vi"("Run VI Named String"=w420, "Multi Run Row"=w419) -> ("Check Meas Setup?"=w418:bool)  [unwired: 1 in, 8 out]
            n161 = Select(t="Check Measurement Setup", s=w418, f=w416) -> (s? t:f=w415:string)
          }
          frame "Set Tunnel Speed Only", Default {
          }
        }
      }
      frame "Check Measurement Setup" {
        n162 = Unbundle By Name(w429) -> ("Meas Setup File"=w427:string)
        n163 = call "Check_Measurement_Setups.vi"("Measurement Setup String"=w427) -> ("Measurement Setup String Out"=w426:string, "Error Comments"=w425:string)
        n164 = Bundle By Name(cluster=w429, "Meas Setup File"=w426) -> (w428:T1)
        n165 = Concatenate Strings(w432, w425) -> (w433:string)
      }
      frame "Check Maximum tunnel speed" {
        n166 = case shown="\"Auto Calibrate\"" w440 {
          tunnel: w437 -> [w462 _]
          tunnel: [w453 FALSE] -> w439
          tunnel: [w452 0.0] -> w438
          frame "Auto Calibrate" {
            n167 = Unbundle By Name(w462) -> ("Specific Arguments"=w461:string)
            n168 = call "Get_array_values_fr_String.vi"("String Value"=w461) -> ("Numeric Array"=w455:dbl[], "String array"=w460:string[])
            n169 = Index Array(array=w460, index=0 ("Index")) -> (element=w458:string)
            n170 = Equal?(x=w458, y="Tunnel Speed" ("Output Array")) -> (x = y?=w453:bool)
            n171 = Array Subset(array=w455, index=1 ("Array Index")) -> (w454:dbl[])  [unwired: 1 in]
            n172 = Array Max & Min(array=w454) -> (max value=w452:dbl)  [unwired: 3 out]
          }
          frame "Set Tunnel Speed Only", Default {
          }
        }
        n173 = case shown="False" w439 {
          tunnel: [w450 w451] -> w447
          tunnel: w437 -> [w449 _]
          tunnel: w438 -> [_ w451]
          frame False {
            n174 = Unbundle By Name(w449) -> ("Tunnel Speed"=w450:dbl)
          }
          frame True {
          }
        }
        n175 = Greater?(x=w447, y="Max Tunnel Speed") -> (0:w445:bool)
        n176 = Not A Number/Path/Refnum?(number/path/refnum=w447) -> (NaN/Path/Refnum?=w446:bool)
        n177 = Compound Arithmetic op=AND(invert w446, w445) -> (w444:bool)
        n178 = case shown="True" w444 {
          tunnel: w443 -> [w465 w467]
          tunnel: [w465 w466] -> w442
          tunnel: "Max Tunnel Speed" -> [_ w469]
          frame False {
          }
          frame True {
            n179 = Format Into String(format string="The maximum allowable tunnel speed is %.2f m/s.\n" ("Format String"), initial string=w467, w469) -> (resulting string=w466:string)  [unwired: 1 in, 1 out]
          }
        }
      }
      frame "Row type specific check" {
        n180 = case shown="\"Check Beam Power\"" w479 {
          tunnel: w476 -> [w490 w499 w503 w507 w512 w517 w524 w531 w542 w550 w564 w570 w675 w680 w684 w721 w773 w801 w806 w810 w822 w826 w832]
          tunnel: [string[] [] string[] [] string[] [] string[] [] w513 w520 w527 w534 w547 w555 w565 w574 w677 string[] [] w701 string[] [] w768 string[] [] string[] [] string[] [] string[] [] string[] [] string[] []] -> w478
          tunnel: [w484 "" "" "" "" "" "" "" w543 w552 "" w568 w671 "" w696 w717 w784 w803 "" w812 "" "" w834] -> w482
          tunnel: [w493 w500 w504 w508 w511 w518 w525 w532 w541 w551 w563 w572 w665 w681 w695 w724 w769 "check entered filename etc" "check entered filename etc" "check entered filename etc" "check entered filename etc" "check entered filename etc" "check entered filename etc"] -> w477
          tunnel: "Check source details" -> [_ w500 w504 _ _ _ _ _ _ _ w563 _ w665 w681 w695 w723 w770 _ _ _ _ _ _]
          tunnel: "Sort out start and end positions" -> [_ _ _ _ _ w518 w525 w532 _ w551 _ w571 _ _ _ _ _ _ _ _ _ _ _]
          tunnel: "Check for Start NaNs" -> [w493 _ _ w508 w511 _ _ _ w541 _ _ w573 _ _ _ _ _ _ _ _ _ _ _]
          tunnel: [w489 w499 w503 w507 w512 w517 w524 w531 w542 w550 w564 w569 w675 w680 w684 w720 w773 w801 w806 w810 w822 w826 w830] -> w471
          tunnel: w470 -> [_ _ _ _ _ _ _ _ _ _ _ _ _ _ _ w726 _ _ _ _ _ _ _]
          frame "Move Traverse Only" {
            n181 = Unbundle By Name(w490) -> ("Specific Arguments"=w491:string)
            n182 = call <vilib>:"Trim Whitespace.vi"("string"=w491) -> ("trimmed string"=w485:string)  [unwired: 1 in]
            n183 = Equal?(x=w485, y="No Backlash") -> (x = y?=w488:bool)
            n184 = Empty String/Path?(string/path=w485) -> (empty?=w487:bool)
            n185 = Or(x=w487, y=w488) -> (x .or. y?=w486:bool)
            n186 = case shown="False" w486 {
              tunnel: w485 -> [w496 _]
              tunnel: [w495 ""] -> w484
              frame False {
                n187 = Format Into String(format string="\"%s\" is an Incorrect Specific Argument. It should either be left blank or say \"No Backlash\"\n", w496) -> (resulting string=w495:string)  [unwired: 2 in, 1 out]
              }
              frame True {
              }
            }
            n188 = Bundle By Name(cluster=w490, "Specific Arguments"=w485) -> (w489:T1)
          }
          frame "Set Tunnel Speed Only" {
          }
          frame "Set Source Only" {
          }
          frame "Set Measurement Conditions" {
          }
          frame "Single Measurement" {
            n189 = Build Array("Averaging:Time:(mins)" ("Label for value"), "Filename:HD:Users" ("Label for value")) -> (w513:string[])
          }
          frame "Vertical Profile" {
            n190 = Build Array("Number:Of:Points" ("Label for value"), "Averaging:Time:(mins)" ("Label for value"), "Filename:HD:Users" ("Label for value")) -> (w520:string[])
          }
          frame "Lateral Profile" {
            n191 = Build Array("Number:Of:Points" ("Label for value"), "Averaging:Time:(mins)" ("Label for value"), "Filename:HD:Users" ("Label for value")) -> (w527:string[])
          }
          frame "Longitudinal Profile" {
            n192 = Build Array("Number:Of:Points" ("Label for value"), "Averaging:Time:(mins)" ("Label for value"), "Filename:HD:Users" ("Label for value")) -> (w534:string[])
          }
          frame "Explore Volume" {
            n193 = Unbundle By Name(w542) -> ("Specific Arguments"=w540:string)
            n194 = Build Array("Averaging:Time:(mins)" ("Label for value"), "Filename:HD:Users" ("Label for value")) -> (w547:string[])
            n195 = Fract/Exp String To Number(string=w540) -> (number=w539:dbl)  [unwired: 4 out]
            n196 = Greater Than 0?(x=w539) -> (x > 0?=w538:bool)
            n197 = Format Into String(format string="\"%s\" is an Incorrect Specific Argument. Please enter the radius of the volume in mm.\n", w540) -> (resulting string=w544:string)  [unwired: 2 in, 1 out]
            n198 = Select(t="", s=w538, f=w544) -> (s? t:f=w543:string)
          }
          frame "Multi-Axis Profile" {
            n199 = Unbundle By Name(w550) -> ("Spacing"=w553:T2)
            n200 = Build Array("Number:Of:Points" ("Label for value"), "Averaging:Time:(mins)" ("Label for value"), "Filename:HD:Users" ("Label for value")) -> (w555:string[])
            n201 = case shown="\"Gauss\"" w553 {
              tunnel: ["" "You are not allowed to specify gaussian spacing for a Multi-Axis profile.\n" "You are not allowed to specify Log spacing for a Multi-Axis profile.\n" "\"N/A\" is not a valid point spacing.\n"] -> w552
              frame "Linear", Default {
              }
              frame "Gauss" {
              }
              frame "Log" {
              }
              frame "N/A" {
              }
            }
          }
          frame "Traverse 3D Volume" {
            n202 = Build Array("Averaging:Time:(mins)" ("Label for value"), "Filename:HD:Users" ("Label for value")) -> (w565:string[])
          }
          frame "Auto Calibrate" {
            n203 = stacked-sequence {
              seq-local: [w577 _ _ _ _] -> [_ _ _ _ w664]
              seq-local: [w576 _ _ _ _] -> [_ w607 _ w653 _]
              seq-local: [w575 _ _ _ _] -> [_ w606 w616 w655 _]
              seq-local: [_ w605 _ _ _] -> [_ _ _ _ w663]
              seq-local: [_ _ w618 _ _] -> [_ _ _ _ w662]
              seq-local: [_ _ _ w646 _] -> [_ _ _ _ w660]
              tunnel: [w586 _ _ _ _] -> w574
              tunnel: w573 -> [w585 _ _ _ _]
              tunnel: [w584 _ _ _ _] -> w572
              tunnel: w571 -> [w583 _ _ _ _]
              tunnel: w570 -> [w582 _ w617 w648 _]
              tunnel: [_ _ w615 _ _] -> w569
              tunnel: [_ _ _ _ w661] -> w568
              frame #0 {
                n204 = Unbundle By Name(w582) -> ("Specific Arguments"=w579:string)
                n205 = call "Get_array_values_fr_String.vi"("String Value"=w579) -> ("Numeric Array"=w576:dbl[], "String array"=w580:string[])
                n206 = Build Array("Tunnel Speed", "Traverse Position", "Concentration") -> (w589:string[])
                n207 = Index Array(array=w580, index=0 ("Index")) -> (element=w578:string)
                n208 = Build Array("Averaging:Time:(mins)" ("Label for value")) -> (w586:string[])
                n209 = Search 1D Array(1D array=w589, element=w578) -> (index of element=w575:i32)  [unwired: 1 out]
                n210 = case shown="0, Default" w575 {
                  tunnel: [w603 w604] -> w584
                  tunnel: w585 -> [w603 _]
                  tunnel: w583 -> [_ w604]
                  frame 0, Default {
                  }
                  frame 1 {
                  }
                }
                n211 = Greater Or Equal To 0?(x=w575) -> (x >= 0?=w587:bool)
                n212 = case shown="False" w587 {
                  tunnel: w589 -> [w594 _]
                  tunnel: [w593 ""] -> w577
                  frame False {
                    n213 = for {
                      shift-right: [w599] -> w596
                      shift-left: "Incorrect Specific Argument. The options are: " -> [w600]
                      tunnel: w594 -> [w601] mode=indexing
                      w598 = "  " ("Substring")
                      n214 = Concatenate Strings(w600, w598, w601, w598) -> (w599:string)
                    }
                    n215 = Concatenate Strings(w596, "\r\n") -> (w593:string)
                  }
                  frame True {
                  }
                }
              }
              frame #1 {
                n216 = Array Size(array=w607) -> (size(s)=w614:i32)
                n217 = Less?(x=w614, y=3) -> (x < y?=w610:bool)
                n218 = Equal To 0?(x=w606) -> (x = 0?=w611:bool)
                n219 = Compound Arithmetic op=AND(w610, w611) -> (w609:bool)
                n220 = Select(t="You need to enter the desired tunnel speeds in the \"Specfic Arguments\" Box   eg.  Tunnel Speed;1;2;3;4\n", s=w609, f="") -> (s? t:f=w605:string)
              }
              frame #2 {
                n221 = global read "Trav_pos_global.vi" "Work in Tunnel Coordinates?"() -> (w629:T7)
                n222 = Unbundle By Name(w617) -> ("Filename"=w622:path)
                n223 = call "Current_Filepath.vi"("Short_Name"="Cal" ("Data Type"), "Filename in"=w622, "Data Type"="Calibrations") -> ("Filename Out"=w620:path)  [unwired: 1 in, 1 out]
                n224 = Equal?(x=w629, y=Tunnel_Coordinates."Work in Model Coordinates" ("Work in Tunnel Coordinates?")) -> (x = y?=w624:bool)
                n225 = Equal?(x=2, y=w616) -> (x = y?=w626:bool)
                n226 = And(x=w624, y=w626) -> (x .and. y?=w625:bool)
                n227 = case shown="True" w625 {
                  tunnel: [w633 w638] -> w621
                  tunnel: w617 -> [w633 w634]
                  frame False {
                  }
                  frame True {
                    n228 = global read "Extra_Commands_Global.vi" "Work in Tunnel Coordinates"() -> (w636:string)
                    n229 = Unbundle By Name(w634) -> ("Extra Commands"=w635:string)
                    n230 = call "Extra_Commands.vi"("String to Search"=w635, "Command"=w636) -> ("Command Found"=w637:bool)  [unwired: 1 in, 4 out]
                    n231 = case shown="False" w637 {
                      tunnel: [w644 w645] -> w638
                      tunnel: w636 -> [w643 _]
                      tunnel: w635 -> [w642 _]
                      tunnel: w634 -> [w640 w645]
                      frame False {
                        n232 = Concatenate Strings(w643, "  " ("string"), w642) -> (w641:string)
                        n233 = Bundle By Name(cluster=w640, "Extra Commands"=w641) -> (w644:T1)
                      }
                      frame True {
                      }
                    }
                  }
                }
                n234 = call "Does_file_exist_(simple).vi"("Pathname"=w620) -> ("exists?"=w632:bool)
                n235 = Select(t="", s=w632, f="The calibration file cannot be found.\n") -> (s? t:f=w618:string)
                n236 = Bundle By Name(cluster=w621, "Filename"=w620) -> (w615:T1)
              }
              frame #3 {
                n237 = Equal?(x=2, y=w655) -> (x = y?=w650:bool)
                n238 = Array Size(array=w653) -> (size(s)=w647:i32)
                n239 = Greater?(x=w647, y=1) -> (0:w651:bool)
                n240 = And(x=w651, y=w650) -> (x .and. y?=w649:bool)
                n241 = case shown="False" w649 {
                  tunnel: w648 -> [_ w659]
                  tunnel: w647 -> [_ _]
                  tunnel: ["" w657] -> w646
                  frame False {
                  }
                  frame True {
                    n242 = Unbundle By Name(w659) -> ("Specific Arguments"=w658:string)
                    n243 = call "Read_FFID_Auto_Calib_Setup.vi"("Specific Argument"=w658) -> ("Error String"=w657:string)  [unwired: 4 out]
                  }
                }
              }
              frame #4 {
                n244 = Concatenate Strings(w664, w663, w662, w660) -> (w661:string)
              }
            }
          }
          frame "Meas Fast FID Bkgnd" {
            n245 = Unbundle By Name(w675) -> ("Specific Arguments"=w670:string)
            n246 = call "Get_array_values_fr_String.vi"("String Value"=w670) -> ("String array"=w669:string[])  [unwired: 1 out]
            n247 = Index Array(array=w669, index=0) -> (element=w667:string)
            n248 = Empty String/Path?(string/path=w667) -> (empty?=w673:bool)
            n249 = Build Array("Averaging:Time:(mins)" ("Label for value")) -> (w677:string[])
            n250 = Equal?(x=w667, y="Use Source Divertor Valve") -> (x = y?=w666:bool)
            n251 = Or(x=w673, y=w666) -> (x .or. y?=w672:bool)
            n252 = case shown="False" w672 {
              tunnel: ["Specific Argument should either be blank or\nUse Source Divertor Valve ; (wait time in seconds optional)" ""] -> w671
              frame False {
              }
              frame True {
              }
            }
          }
          frame "Check Beam Power" {
          }
          frame "Scanning Valve Measurement" {
            w697 = ext -0.5  # lo
            w698 = ext 47.5  # hi
            n253 = Unbundle By Name(w684) -> ("Specific Arguments"=w694:string)
            n254 = call "Get_array_values_fr_String.vi"("String Value"=w694) -> ("Numeric Array"=w693:dbl[], "String array"=w689:string[])
            n255 = Build Array("Averaging:Time:(mins)" ("Label for value"), "Filename:HD:Users" ("Label for value")) -> (w701:string[])
            n256 = Index Array(array=w689, index=0) -> (element=w688:string)
            n257 = Empty String/Path?(string/path=w688) -> (empty?=w686:bool)
            n258 = Index Array(array=w693, index=0) -> (element=w691:dbl)
            n259 = In Range and Coerce(upper limit=w698, x=w691, lower limit=w697) -> (In Range?=w687:bool)  [unwired: 1 out]
            n260 = Compound Arithmetic op=AND(invert w686, w687) -> (w685:bool)
            n261 = Select(t="", s=w685, f="Enter the scanning valve port number between 0 and 47 in the specific arguments box.\n") -> (s? t:f=w696:string)
          }
          frame "Set ADAM Ch" {
            n262 = Unbundle By Name(w721) -> ("Specific Arguments"=w728:string, "Extra Commands"=w716:string)
            n263 = while {
              shift-right: [w762] -> w727
              shift-left: _ -> [w755]
              shift-right: [w761] -> _
              shift-left: _ -> [w760]
              tunnel: w726 -> [w761]
              stop <- TRUE stop-if-true
              n264 = Array Size(array=w755) -> (size(s)=w759:i32)
              n265 = Less?(x=w761, y=w760) -> (x < y?=w757:bool)
              n266 = Equal To 0?(x=w759) -> (x = 0?=w758:bool)
              n267 = Or(x=w758, y=w757) -> (x .or. y?=w756:bool)
              n268 = case shown="True" w756 {
                tunnel: [w763 w764] -> w762
                tunnel: w755 -> [w763 _]
                frame False {
                }
                frame True {
                  n269 = call "Get_ADAM_Ch_names_client.vi"("Channel names set"=Channel_names."Active + Off") -> ("Ch names"=w764:string[])
                }
              }
            }
            n270 = call "Get_array_values_fr_String.vi"("String Value"=w716) -> ("Numeric Array"=w712:dbl[])  [unwired: 1 out]
            n271 = call "Get_array_values_fr_String.vi"("String Value"=w728) -> ("String array"=w713:string[])  [unwired: 1 out]
            n272 = for {
              tunnel: w727 -> [w736]
              tunnel: w713 -> [w735] mode=indexing
              tunnel: w712 -> [w731]
              tunnel: [w733] -> w715 mode=indexing
              tunnel: [w732] -> w714 mode=indexing
              i -> [w730]
              n273 = Index Array(array=w731, index=w730) -> (element=w734:dbl)
              n274 = Search 1D Array(1D array=w736, element=w735) -> (index of element=w737:i32)  [unwired: 1 out]
              n275 = Not A Number/Path/Refnum?(number/path/refnum=w734) -> (NaN/Path/Refnum?=w732:bool)
              n276 = Greater Or Equal To 0?(x=w737) -> (x >= 0?=w733:bool)
            }
            n277 = Array Size(array=w713) -> (size(s)=w707:i32)
            n278 = Array Size(array=w712) -> (size(s)=w711:i32)
            n279 = Not Equal?(x=w707, y=w711) -> (x != y?=w709:bool)
            n280 = Greater Than 0?(x=w707) -> (x > 0?=w705:bool)
            n281 = Or Array Elements(Boolean array=w714) -> (logical OR=w710:bool)
            n282 = And Array Elements(Boolean array=w715) -> (logical AND=w706:bool)
            n283 = Or(x=w709, y=w710) -> (x .or. y?=w708:bool)
            n284 = Select(t="You have not specified a Value to Set the ADAM channel to.\nPlease give the values separated by ; in the Extra Commands string", s=w708, f="") -> (s? t:f=w717:string)
            n285 = And(x=w705, y=w706) -> (x .and. y?=w704:bool)
            n286 = case shown="True" w704 {
              tunnel: w727 -> [w748 _]
              tunnel: w713 -> [w740 w750]
              tunnel: w726 -> [w746 _]
              tunnel: [w744 FALSE ("Cancel")] -> w725
              tunnel: w721 -> [w742 w752]
              tunnel: [w741 w751] -> w720
              frame False {
                n287 = Format Into String(format string="Please Select the ADAM Channels that you want to set in row %d", w746) -> (resulting string=w745:string)  [unwired: 2 in, 1 out]
                n288 = call "Select_Strings.vi"("Available Ch names"=w748, "Message"=w745, "Selector mode"=T8."One or more", "Desired Ch names (in)"=w740) -> ("Cancel"=w744:bool, "Selected Channel Names"=w739:string[])  [unwired: 1 in, 2 out]
                n289 = call "Put_Array_into_String.vi"("String array"=w739) -> ("String Value"=w738:string)
                n290 = Bundle By Name(cluster=w742, "Specific Arguments"=w738) -> (w741:T1)
              }
              frame True {
                n291 = call "Put_Array_into_String.vi"("String array"=w750) -> ("String Value"=w749:string)
                n292 = Bundle By Name(cluster=w752, "Specific Arguments"=w749) -> (w751:T1)
              }
            }
            n293 = Select(t="Close Front Panel", s=w725, f=w723) -> (s? t:f=w724:string)
          }
          frame "Run VI Named:" {
            w778 = "Run_VI_Named_specific.vi"
            n294 = Unbundle By Name(w773) -> ("Specific Arguments"=w781:string)
            n295 = global read "Constants_global.vi" "Run VI Folder"() -> (w779:path)
            n296 = Match Pattern(string=w781, regular expression=";") -> (before substring=w782:string)  [unwired: 4 out]
            n297 = call <vilib>:"Trim Whitespace.vi"("string"=w782) -> ("trimmed string"=w774:string)  [unwired: 1 in]
            n298 = call "Run_VI_Named_specific.vi"("Run VI Named String"=w774, "Earlier Filenames"="Earlier Filenames", "Multi Run Row"=w773) -> ("Checks"=w768:string[], "Error String"=w767:string, "Check for start NaNs?"=w772:bool)  [unwired: 6 out]
            n299 = Select(t="Check for Start NaNs" ("Label for value"), s=w772, f=w770) -> (s? t:f=w769:string)
            n300 = Build Path(base path=w779, name or relative path=w774) -> (appended path=w785:path)
            n301 = Not Equal?(x=w774, y=w778) -> (x != y?=w777:bool)
            n302 = call "Does_file_exist_(simple).vi"("Pathname"=w785) -> ("exists?"=w776:bool)
            n303 = And(x=w776, y=w777) -> (x .and. y?=w775:bool)
            n304 = case shown="False" w775 {
              tunnel: [w792 ""] -> w780
              tunnel: w779 -> [w788 _]
              tunnel: w778 -> [w786 _]
              frame False {
                w790 = "\r\n"
                n305 = Build Array(w786) -> (w787:string[])
                n306 = call "List_files_in_order_of_age.vi"("Files to Hide"=w787, "Folder"=w788) -> ("file names"=w789:string[])
                n307 = for {
                  shift-right: [w796] -> w793
                  shift-left: "Cannot find the VI to run. Specific Argument options are:" -> [w797]
                  tunnel: w789 -> [w798] mode=indexing
                  w795 = "  " ("Substring")
                  n308 = Concatenate Strings(w797, w795, w798, w795) -> (w796:string)
                }
                n309 = Concatenate Strings(w793, w790, "Please place one of these strings in the \"Specific Argument\" field.", w790) -> (w792:string)
              }
              frame True {
              }
            }
            n310 = Concatenate Strings(w767, w780) -> (w784:string)
          }
          frame "Wait (minutes)" {
            n311 = Unbundle By Name(w801) -> ("Specific Arguments"=w802:string)
            n312 = call "Wait_Case_Arg.vi"("Specific Argument"=w802) -> ("Error Comments"=w803:string)  [unwired: 1 in, 4 out]
          }
          frame "Send Message" {
          }
          frame "Synchronize With:" {
            n313 = local read "Current Sync Number"() -> (w811:i32)
            n314 = call "Synchronize_Prog_Arg.vi"("Execution Row"=w810) -> ("Error Comments"=w813:string, "Sync No"=w819:i32)  [unwired: 3 out]
            n315 = Format Into String(format string="This should be Synchroisation number %d.\n" ("Format String"), w811) -> (resulting string=w816:string)  [unwired: 2 in, 1 out]
            n316 = Equal?(x=w819, y=w811) -> (x = y?=w818:bool)
            n317 = Select(t="", s=w818, f=w816) -> (s? t:f=w814:string)
            n318 = Concatenate Strings(w814, w813) -> (w812:string)
          }
          frame "Fall Back to this Row" {
          }
          frame "Turn Off Row Repeating" {
          }
          frame "Blank Row" {
            n319 = Unbundle By Name(w832) -> ("Comments"=w838:string)
            n320 = Match Pattern(string=w838, regular expression="(No Match Info)") -> (before substring=w831:string, after substring=w835:string)  [unwired: 3 out]
            n321 = Empty String/Path?(string/path=w835) -> (empty?=w836:bool)
            n322 = Bundle By Name(cluster=w832, "Comments"=w831) -> (w830:T1)
            n323 = Select(t=w835, s=w836, f="The Row Type Selector \"%s\" was not matched. Please select the desired type.\n") -> (s? t:f=w834:string)
          }
        }
        "Checks" <- w478
        n324 = Concatenate Strings(w481, w482) -> (w480:string)
      }
      frame "Sort out start and end positions" {
        n325 = Unbundle By Name(w846) -> ("Start X"=w858:sgl, "Start Y"=w857:sgl, "Start Z"=w856:sgl, "End X"=w855:sgl, "End Y"=w854:sgl, "End Z"=w853:sgl, "Extra Commands"=w842:string)
        n326 = call "Which_Trav_Setup.vi"("Extra Command String"=w842) -> ("Traverse Setups"=w840:string[])
        n327 = Build Array(w858, w857, w856) -> (w849:sgl[])
        n328 = Build Array(w855, w854, w853) -> (w848:sgl[])
        n329 = Index Array(array=w840) -> (element=w841:string)  [unwired: 1 in]
        n330 = call "Rig_Pict_Display_Pref.vi"("Traverse Name"=w841) -> ("Which Axis is vertical?"=w852:enum16{"X Axis", "Y Axis", "Z Axis"})  [unwired: 7 out]
        n331 = case shown="\"Longitudinal Profile\"" w847 {
          tunnel: [w898 FALSE w914 w927 FALSE] -> w861
          tunnel: [w897 FALSE w913 w926 FALSE] -> w860
          tunnel: [w896 FALSE w912 w925 FALSE] -> w859
          tunnel: w852 -> [w895 _ w911 w924 _]
          frame "Vertical Profile" {
            n332 = case shown="\"Z Axis\"" w895 {
              tunnel: [FALSE TRUE TRUE] -> w898
              tunnel: [TRUE FALSE TRUE] -> w897
              tunnel: [TRUE TRUE FALSE] -> w896
              frame "X Axis" {
              }
              frame "Y Axis" {
              }
              frame "Z Axis" {
              }
            }
          }
          frame "Auto Calibrate" {
          }
          frame "Lateral Profile" {
            n333 = case shown="\"Y Axis\"" w911 {
              tunnel: [TRUE TRUE TRUE] -> w914
              tunnel: [TRUE TRUE FALSE] -> w913
              tunnel: [FALSE FALSE TRUE] -> w912
              frame "X Axis" {
              }
              frame "Y Axis" {
              }
              frame "Z Axis" {
              }
            }
          }
          frame "Longitudinal Profile" {
            n334 = case shown="\"Y Axis\"" w924 {
              tunnel: [FALSE FALSE FALSE] -> w927
              tunnel: [TRUE TRUE TRUE] -> w926
              tunnel: [TRUE TRUE TRUE] -> w925
              frame "X Axis" {
              }
              frame "Y Axis" {
              }
              frame "Z Axis" {
              }
            }
          }
          frame "Multi-Axis Profile", Default {
          }
        }
        n335 = Build Array(w861, w860, w859) -> (w850:bool[])
        "Fixed Axis" <- w850
        n336 = for {
          tunnel: w850 -> [w868] mode=indexing
          tunnel: w849 -> [w867] mode=indexing
          tunnel: w848 -> [w866] mode=indexing
          shift-right: [w863] -> w845
          shift-left: w846 -> [w864]
          i -> [w865]
          n337 = case shown="True" w868 {
            tunnel: w867 -> [_ w874]
            tunnel: w866 -> [_ w873]
            tunnel: w865 -> [_ w872]
            tunnel: w864 -> [w869 w871]
            tunnel: [w869 w870] -> w863
            frame False {
            }
            frame True {
              n338 = Not A Number/Path/Refnum?(number/path/refnum=w874) -> (NaN/Path/Refnum?=w875:bool)
              n339 = Not A Number/Path/Refnum?(number/path/refnum=w873) -> (NaN/Path/Refnum?=w877:bool)
              n340 = Exclusive Or(1:w877, 2:w875) -> (0:w876:bool)
              n341 = case shown="True" w876 {
                tunnel: w875 -> [_ w885]
                tunnel: w874 -> [_ w884]
                tunnel: w873 -> [_ w883]
                tunnel: w872 -> [_ w882]
                tunnel: w871 -> [w878 w881]
                tunnel: [w878 w880] -> w870
                frame False {
                }
                frame True {
                  n342 = Select(t=w883, s=w885, f=w884) -> (s? t:f=w879:sgl)
                  n343 = case shown="2" w882 {
                    tunnel: w881 -> [w888 w891 w894]
                    tunnel: [w887 w890 w893] -> w880
                    tunnel: w879 -> [w886 w889 w892]
                    frame 0, Default {
                      n344 = Bundle By Name(cluster=w888, "Start X"=w886, "End X"=w886) -> (w887:T1)
                    }
                    frame 1 {
                      n345 = Bundle By Name(cluster=w891, "Start Y"=w889, "End Y"=w889) -> (w890:T1)
                    }
                    frame 2 {
                      n346 = Bundle By Name(cluster=w894, "Start Z"=w892, "End Z"=w892) -> (w893:T1)
                    }
                  }
                }
              }
            }
          }
        }
      }
      frame "Check for position NaNs" {
        n347 = global read "Extra_Commands_Global.vi" "Skip Traverse Position Demand"() -> (w943:string)
        n348 = Unbundle By Name(w946) -> ("Extra Commands"=w942:string, "Start X"=w955:sgl, "Start Y"=w953:sgl, "Start Z"=w954:sgl, "End X"=w952:sgl, "End Y"=w951:sgl, "End Z"=w950:sgl)
        n349 = call "Extra_Commands.vi"("String to Search"=w942, "Command"=w943) -> ("Command Found"=w940:bool)  [unwired: 1 in, 4 out]
        n350 = case shown="False" w940 {
          tunnel: w955 -> [w970 _]
          tunnel: w954 -> [w969 _]
          tunnel: w953 -> [w968 _]
          tunnel: w952 -> [w967 _]
          tunnel: w951 -> [w966 _]
          tunnel: w950 -> [w965 _]
          tunnel: [w961 w971] -> w949
          tunnel: [w960 TRUE] -> w948
          tunnel: "" -> [w959 w971]
          frame False {
            n351 = Build Array(w970, w968, w969, w967, w966, w965) -> (w964:sgl[])
            n352 = Not A Number/Path/Refnum?(number/path/refnum=w964) -> (NaN/Path/Refnum?=w963:bool[])
            n353 = Or Array Elements(Boolean array=w963) -> (logical OR=w960:bool)
            n354 = Select(t="Some of the Start and End positions are NaN.\n" ("f"), s=w960, f=w959) -> (s? t:f=w961:string)
          }
          frame True {
          }
        }
        n355 = case shown="\"Set Tunnel Speed Only\", Default" w944 {
          tunnel: w948 -> [_ w977]
          tunnel: ["Check source details" ("t") w976] -> w947
          frame "Multi-Axis Profile" {
          }
          frame "Set Tunnel Speed Only", Default {
            n356 = Select(t="Check source details", s=w977, f="Check profile rows") -> (s? t:f=w976:string)
          }
        }
        n357 = Concatenate Strings(w957, w949) -> (w956:string)
      }
      frame "Check for Start NaNs" {
        n358 = Unbundle By Name(w983) -> ("Extra Commands"=w979:string, "Start X"=w988:sgl, "Start Y"=w986:sgl, "Start Z"=w987:sgl)
        n359 = global read "Extra_Commands_Global.vi" "Skip Traverse Position Demand"() -> (w980:string)
        n360 = call "Extra_Commands.vi"("String to Search"=w979, "Command"=w980) -> ("Command Found"=w978:bool)  [unwired: 1 in, 4 out]
        n361 = case shown="True" w978 {
          tunnel: w988 -> [w1000 _]
          tunnel: w987 -> [w999 _]
          tunnel: w986 -> [w998 _]
          tunnel: "" -> [w995 w1001]
          tunnel: [w993 w1001] -> w984
          frame False {
            n362 = Build Array(w1000, w998, w999) -> (w997:sgl[])
            n363 = Not A Number/Path/Refnum?(number/path/refnum=w997) -> (NaN/Path/Refnum?=w996:bool[])
            n364 = Or Array Elements(Boolean array=w996) -> (logical OR=w992:bool)
            n365 = Select(t="Some of the Start coordinates are NaN.\n" ("f"), s=w992, f=w995) -> (s? t:f=w993:string)
          }
          frame True {
          }
        }
        n366 = Concatenate Strings(w990, w984) -> (w989:string)
      }
      frame "Check profile rows" {
        n367 = Unbundle By Name(w1011) -> ("Start X"=w1033:sgl, "Start Y"=w1032:sgl, "Start Z"=w1031:sgl, "End X"=w1030:sgl, "End Y"=w1029:sgl, "End Z"=w1028:sgl, "Specific Arguments"=w1022:string, "Spacing"=w1017:T2, "No. of pts."=w1016:i32)
        n368 = local read "Fixed Axis"() -> (w1015:bool[])
        n369 = Build Array(w1033, w1032, w1031) -> (w1013:sgl[])
        n370 = Build Array(w1030, w1029, w1028) -> (w1014:sgl[])
        n371 = case shown="\"Specified\"" w1017 {
          tunnel: w1022 -> [_ _ _ _ w1068]
          tunnel: ["" w1041 "\"N/A\" is not a valid point spacing.\n" "" w1063] -> w1021
          tunnel: w1016 -> [_ _ _ _ w1067]
          tunnel: w1015 -> [_ w1039 _ _ _]
          tunnel: w1014 -> [_ w1046 _ _ _]
          tunnel: w1013 -> [_ w1045 _ _ _]
          frame "Linear" {
          }
          frame "Log" {
            n372 = for {
              tunnel: w1046 -> [w1050] mode=indexing
              tunnel: w1045 -> [w1049] mode=indexing
              tunnel: [w1048] -> w1044 mode=indexing
              tunnel: w1039 -> [w1047] mode=indexing
              n373 = case shown="False" w1047 {
                tunnel: w1050 -> [w1056 _]
                tunnel: w1049 -> [w1055 _]
                tunnel: [w1051 FALSE] -> w1048
                frame False {
                  w1054 = 0.001 ("y")
                  n374 = Less?(x=w1056, y=w1054) -> (x < y?=w1052:bool)
                  n375 = Less?(x=w1055, y=w1054) -> (x < y?=w1053:bool)
                  n376 = Or(x=w1052, y=w1053) -> (x .or. y?=w1051:bool)
                }
                frame True {
                }
              }
            }
            n377 = Or Array Elements(Boolean array=w1044) -> (logical OR=w1043:bool)
            n378 = Select(t="For log spacing, Start & End positions must be greater than 0.0001.", s=w1043, f="") -> (s? t:f=w1041:string)
          }
          frame "N/A" {
          }
          frame "Gauss" {
          }
          frame "Specified" {
            n379 = call "Get_array_values_fr_String.vi"("String Value"=w1068) -> ("Numeric Array"=w1062:dbl[])  [unwired: 1 out]
            n380 = Array Size(array=w1062) -> (size(s)=w1061:i32)
            n381 = Decrement(x=w1061) -> (x-1=w1060:i32)
            n382 = Equal?(x=w1060, y=w1067) -> (x = y?=w1066:bool)
            n383 = Select(t="", s=w1066, f="The No of points and No of Arguments do not match.\n") -> (s? t:f=w1063:string)
          }
        }
        n384 = for {
          tunnel: w1015 -> [w1074] mode=indexing
          tunnel: w1013 -> [w1073] mode=indexing
          tunnel: w1014 -> [w1072] mode=indexing
          tunnel: [w1071] -> w1027 mode=indexing
          shift-right: [w1069] -> w1006
          shift-left: bool[] [] -> [w1070]
          n385 = case shown="False" w1074 {
            tunnel: w1073 -> [w1078 w1084]
            tunnel: w1072 -> [w1079 w1083]
            tunnel: [TRUE w1082] -> w1071
            tunnel: w1070 -> [w1076 w1081]
            tunnel: [w1075 w1081] -> w1069
            frame False {
              n386 = Not Equal?(x=w1078, y=w1079) -> (x != y?=w1077:bool)
              n387 = Build Array (concatenate)(w1076, w1077) -> (w1075:bool[])
            }
            frame True {
              n388 = Equal?(x=w1084, y=w1083) -> (x = y?=w1082:bool)
            }
          }
        }
        n389 = Array Size(array=w1006) -> (size(s)=w1005:i32)
        n390 = And Array Elements(Boolean array=w1027) -> (logical AND=w1026:bool)
        n391 = Or Array Elements(Boolean array=w1006) -> (logical OR=w1003:bool)
        n392 = Not Equal To 0?(x=w1005) -> (x != 0?=w1004:bool)
        n393 = And(x=w1003, y=w1004) -> (x .and. y?=w1002:bool)
        n394 = call "Create_Pos_array.vi"("Traverse line"=w1011) -> ("Traverse line Out"=w1010:T1, "Error Messages"=w1009:string)  [unwired: 7 out]
        n395 = Select(t="", s=w1026, f="This profile moves more than one axis.\n") -> (s? t:f=w1023:string)
        n396 = Select(t="", s=w1002, f="The start and end points are the same for this profile.\n") -> (s? t:f=w1019:string)
        n397 = Concatenate Strings(w1009, w1019, w1023, w1021) -> (w1036:string)
        n398 = Concatenate Strings(w1035, w1036) -> (w1034:string)
      }
      frame "Check source details" {
        n399 = Unbundle By Name(w1093) -> ("Carrier_1 Q (l/min)"=w1087:dbl, "Carrier_2 Q (l/min)"=w1086:dbl)  [unwired: 1 out]
        n400 = Add(x=w1087, y=w1086) -> (x+y=w1085:dbl)
        n401 = Greater Than 0?(x=w1085) -> (x > 0?=w1091:bool)
        n402 = Select(t="Check source detail 2", s=w1091, f="check entered filename etc") -> (s? t:f=w1089:string)
      }
      frame "Check source detail 2" {
        n403 = Unbundle By Name(w1104) -> ("Trace Gas Concentration (%)"=w1105:dbl)
        n404 = In Range and Coerce(upper limit=ext 2.1099999999999999999 ("hi"), x=w1105, lower limit=ext 0.0 ("lo")) -> (In Range?=w1099:bool)  [unwired: 1 out]
        n405 = Select(t="", s=w1099, f="The Trace Gas Concentration must be within the range of 0 to 2.1%.\n") -> (s? t:f=w1096:string)
        n406 = Concatenate Strings(w1107, w1096) -> (w1106:string)
      }
      frame "check entered filename etc" {
        n407 = local read "Checks"() -> (w1120:string[])
        n408 = for {
          tunnel: w1120 -> [w1127] mode=indexing
          tunnel: [w1132] -> w1121 mode=indexing
          tunnel: w1117 -> [w1131]
          shift-right: [w1129] -> w1111
          shift-left: w1112 -> [w1130]
          tunnel: [w1128] -> w1110 mode=indexing
          n409 = case shown="\"Filename:HD:Users\"" w1127 {
            tunnel: w1130 -> [w1134 w1142 w1166 w1178]
            tunnel: [w1135 w1145 w1172 w1174] -> w1132
            tunnel: w1131 -> [_ _ _ _]
            tunnel: [w1134 w1142 w1164 w1178] -> w1129
            tunnel: [TRUE ("cancelled") TRUE ("cancelled") w1159 TRUE ("cancelled")] -> w1128
            tunnel: w1127 -> [_ _ _ w1176]
            frame "Number:Of:Points" {
              n410 = Unbundle By Name(w1134) -> ("No. of pts."=w1137:i32)
              n411 = Greater?(x=w1137, y=0) -> (0:w1139:bool)
              n412 = Select(t="", s=w1139, f="For a profile the number of points should be more than 0.\n" ("Format String")) -> (s? t:f=w1135:string)
            }
            frame "Averaging:Time:(mins)" {
              n413 = Unbundle By Name(w1142) -> ("Averaging time (min)"=w1144:dbl)
              n414 = Greater Than 0?(x=w1144) -> (x > 0?=w1143:bool)
              n415 = Select(t="", s=w1143, f="The averaging time should be greater than zero.\n" ("Format String")) -> (s? t:f=w1145:string)
            }
            frame "Filename:HD:Users" {
              w1173 = FALSE  # Show Error handler
              n416 = Unbundle By Name(w1166) -> ("Filename"=w1150:path, "Row No"=w1161:i32, "Row Type Selector"=w1157:T3)
              n417 = call "Row_type_selector_string.vi"("Mode"=w1157) -> ("Output string"=w1156:string)
              n418 = call "Current_Filepath.vi"("Short_Name"="Res" ("Data Type"), "Filename in"=w1150, "Data Type"="Results") -> ("Filename Out"=w1151:path)  [unwired: 1 in, 1 out]
              n419 = Path To String(path=w1151) -> (string=w1170:string)
              n420 = Not A Number/Path/Refnum?(number/path/refnum=w1151) -> (NaN/Path/Refnum?=w1154:bool)
              n421 = Match Pattern(string=w1170, regular expression="-------" ("f")) -> (match substring=w1169:string)  [unwired: 4 out]
              n422 = Empty String/Path?(string/path=w1169) -> (empty?=w1155:bool)
              n423 = Format Into String(format string=" For Row  %d %s." ("Comment"), w1161, w1156) -> (resulting string=w1160:string)  [unwired: 2 in, 1 out]
              n424 = Compound Arithmetic op=AND(w1155, invert w1154) -> (w1153:bool)
              n425 = Select(t=w1151, s=w1153, f=path "") -> (s? t:f=w1168:path)
              n426 = call "Results_filename_checker.vi"("Filelength"=45, "Warn if Already Exists"=FALSE, "Comment"=w1160, "Show Error handler"=w1173, "Results file"=w1168) -> ("Error String"=w1172:string, "cancelled"=w1163:bool, "Results file output"=w1165:path)  [unwired: 1 out]
              n427 = Bundle By Name(cluster=w1166, "Filename"=w1165) -> (w1164:T1)
              n428 = Not(x=w1163) -> (.not. x?=w1159:bool)
            }
            frame "No Match", Default {
              n429 = Concatenate Strings(w1176, " Has not been programmed.\n" ("string")) -> (w1174:string)
            }
          }
        }
        n430 = local read "Edited Row"() -> (w1114:bool)
        n431 = And Array Elements(Boolean array=w1110) -> (logical AND=w1109:bool)
        n432 = Concatenate Strings(w1121) -> (w1119:string)
        n433 = Concatenate Strings(w1118, w1119) -> (w1113:string)
        n434 = Empty String/Path?(string/path=w1113) -> (empty?=w1116:bool)
        n435 = case shown="False" w1116 {
          tunnel: ["Open Front Panel" w1125] -> w1115
          tunnel: w1114 -> [_ w1126]
          frame False {
          }
          frame True {
            n436 = Select(t="Close Front Panel", s=w1126, f="End") -> (s? t:f=w1125:string)
          }
        }
      }
      frame "Open Front Panel" {
        w1183 = TRUE  # Front Panel Window:Open
        n437 = Current VI's Path() -> (path=w1184:path)
        n438 = call "Open_Close_Front_Panel.ph.vi"("Front Panel Window:Open"=w1183, "VI path"=w1184) -> ()  [unwired: 2 out]
        n439 = local write "Edited Row"(TRUE ("Editted Row")) -> ()
        n440 = local write "Execution Row"(w1180) -> ()
      }
      frame "What to do next?" {
        w1192 = ""
        w1191 = "[\r\n]"
        n441 = local read "Execution Row"() -> (w1190:T1)
        n442 = Unbundle By Name(w1190) -> ("Row Type Selector"=w1204:T3, "Specific Arguments"=w1199:string, "Extra Commands"=w1197:string)
        n443 = Wait Until Next ms Multiple(millisecond multiple=u32 100) -> ()  [unwired: 1 out]
        n444 = Not Equal?(x=Multi_run_mode."Blank Row" ("Mode"), y=w1204) -> (x != y?=w1200:bool)
        n445 = call "Replace_Character.vi"("Replace with"=w1192, "Input String"=w1199, "Search For"=w1191) -> ("Output string"=w1198:string)  [unwired: 1 out]
        n446 = call "Replace_Character.vi"("Replace with"=w1192, "Input String"=w1197, "Search For"=w1191) -> ("Output string"=w1196:string)  [unwired: 1 out]
        n447 = Compound Arithmetic op=OR("Edit in Excel", "OK") -> (w1201:bool)
        n448 = Bundle By Name(cluster=w1190, "Specific Arguments"=w1198, "Extra Commands"=w1196) -> (w1188:T1)
        n449 = Compound Arithmetic op=AND(w1201, w1200) -> (w1194:bool)
        n450 = Not Equal?(x=w1188, y=w1190) -> (x != y?=w1189:bool)
        n451 = Not(x="Edit in Excel") -> (.not. x?=w1187:bool)
        n452 = case shown="True" w1189 {
          tunnel: w1188 -> [_ w1208]
          frame False {
          }
          frame True {
            n453 = local write "Execution Row"(w1208) -> ()
          }
        }
        n454 = case shown="True" w1187 {
          tunnel: ["Close Front Panel" w1213] -> w1193
          tunnel: w1194 -> [_ w1212]
          frame False {
          }
          frame True {
            n455 = Select(t="Clean Up Row", s=w1212, f="What to do next?") -> (s? t:f=w1213:string)
          }
        }
        "Error Comments" <- w1195
      }
      frame "Clean Up Row" {
        n456 = call "Traverse_Control_Ch_Names.vi"("Mode"=T4."All Channel Names") -> ("Channel names"=w1222:string[])  [unwired: 1 in]
        n457 = call "Trav_Cluster_to_Row.vi"("Traverse line in"=w1217, "Row Number"=w1218, "Channel names"=w1222) -> ("Traverse line Out"=w1220:T1)  [unwired: 4 out]
      }
      frame "Close Front Panel" {
        w1226 = FALSE  # Front Panel Window:Open
        n458 = Current VI's Path() -> (path=w1227:path)
        n459 = call "Open_Close_Front_Panel.ph.vi"("Front Panel Window:Open"=w1226, "VI path"=w1227) -> ()  [unwired: 2 out]
      }
      frame "End" {
        n460 = local read "Edited Row"() -> (w1235:bool)
        n461 = case shown="True" w1235 {
          tunnel: w1234 -> [w1238 w1241]
          tunnel: [w1238 w1240] -> w1232
          tunnel: w1233 -> [_ w1239]
          frame False {
          }
          frame True {
            n462 = call "Traverse_Control_Ch_Names.vi"("Mode"=T4."All Channel Names") -> ("Channel names"=w1242:string[])  [unwired: 1 in]
            n463 = call "Trav_Cluster_to_Row.vi"("Traverse line in"=w1241, "Row Number"=w1239, "Channel names"=w1242) -> ("Traverse line Out"=w1240:T1)  [unwired: 4 out]
          }
        }
        n464 = local write "Error Comments"(w1236) -> ()
      }
    }
    "Traverse line Out" <- w8
  }
  "Execution Row Out" <- w2
  "Continue?" <- w1
